vi "Update_Current_Value_client.vi"(0 "Don't Bother with check?":bool, 1 "Update array in":T1[](array[typedef]) {"New Value" format="%.2f"}) -> ()   [LabVIEW 2017]
doc: "This is an example of using features of the VI Server as a client. It shows how you might browse from one or more applications that may be exporting data from one or more data stations. \n\nThe example shows how to query a server for its list of exported VIs, how to get references to the VIs, and how call them with the Call By Reference function."
uses:
  Sub VIs/ADAM Controls/Update_scan_value.ctl
  Anemometry/Anemometry Sub Vis/Controls/Global_mode.ctl
  Anemometry/Anemometry Sub Vis/Globals/Preference_global.vi
panel:
  in  "Server type":refnum<vi>
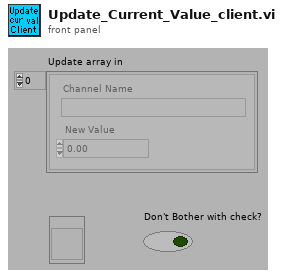
[diagram p1: front panel]
types:
  T1 = typedef "Update_scan_value.ctl" = cluster{"Channel Name":string, "New Value":dbl}
  T2 = typedef "Server_Comms.ctl" = enum16{"Server Link Healthy", "Do Not Link To Server"}
  T3 = typedef "Global_mode.ctl" = enum16{"Read Global", "Load Global From File", "Write Global to File"}
  T4 = enum16{"Append to Global", "Read Global then Clear"}
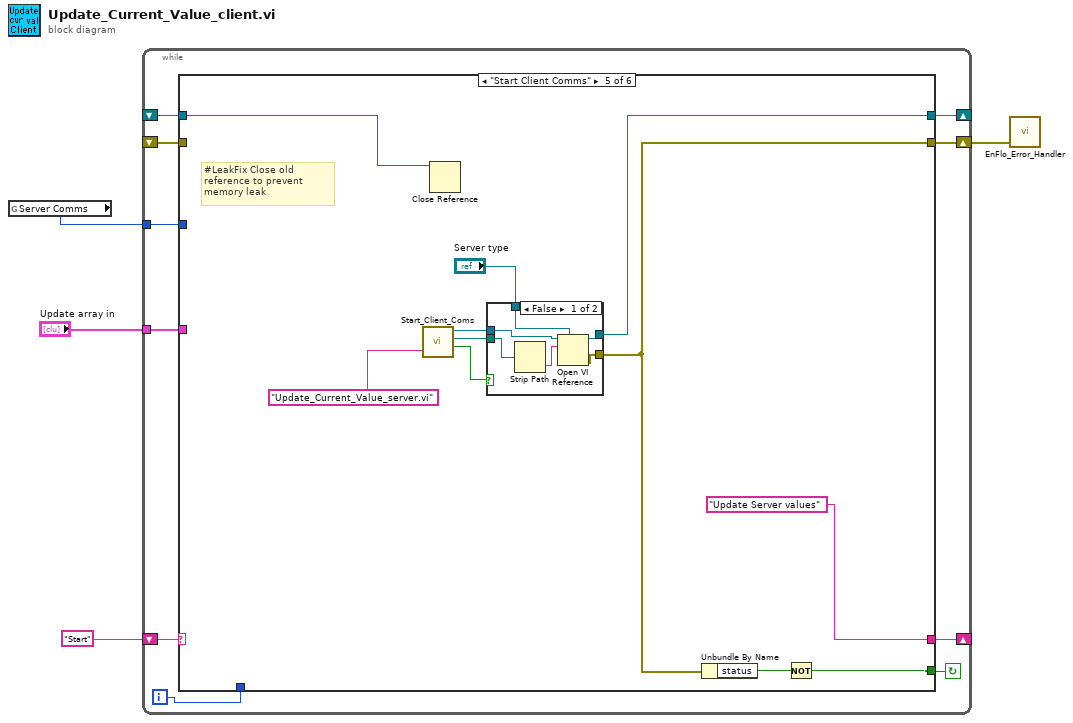
[diagram p0: block diagram]
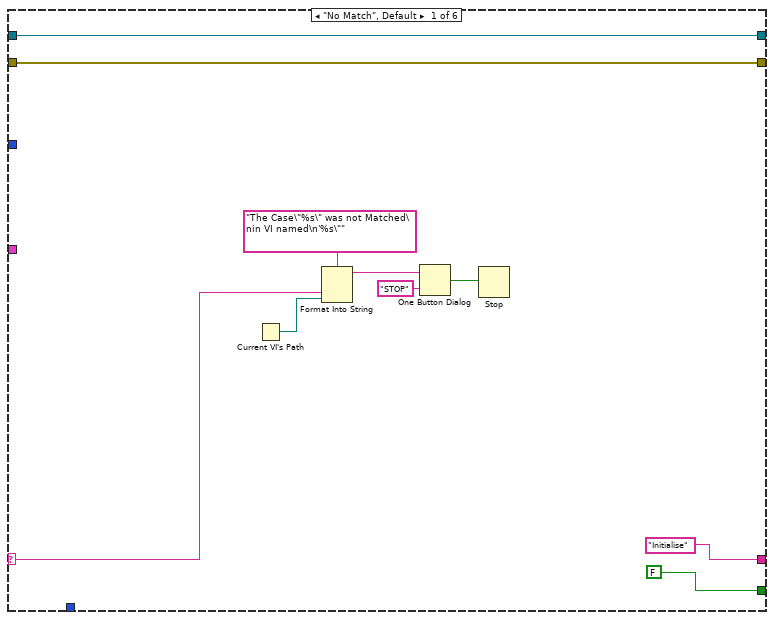
[diagram p2: hidden frame]
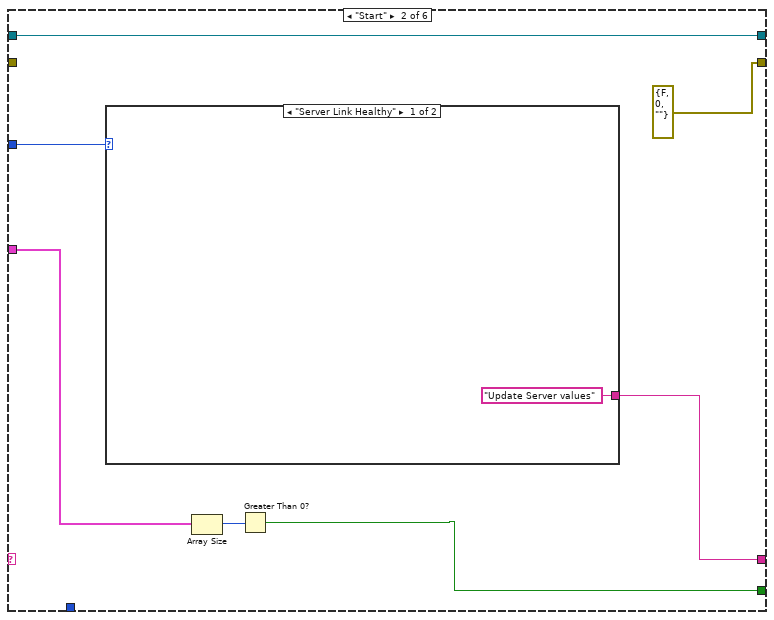
[diagram p3: hidden frame]
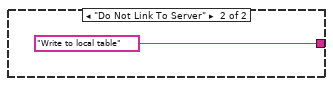
[diagram p4: hidden frame]
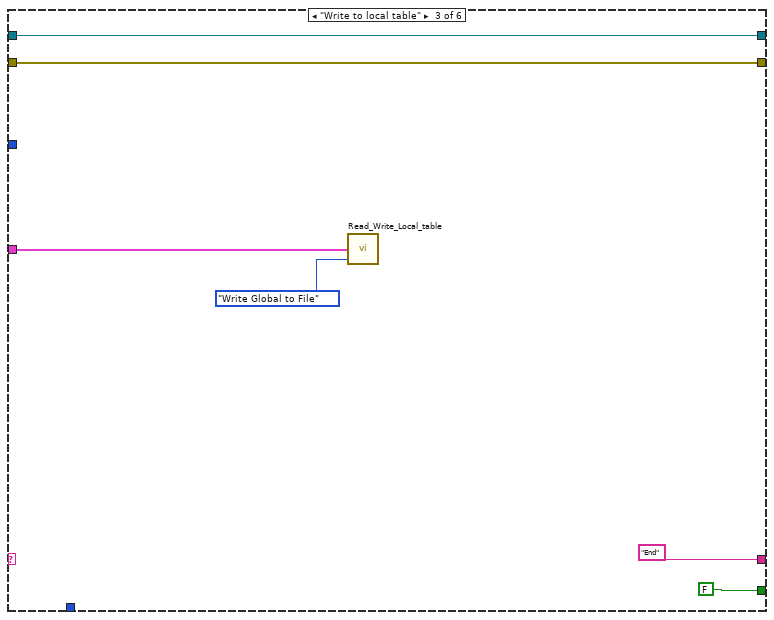
[diagram p5: hidden frame]
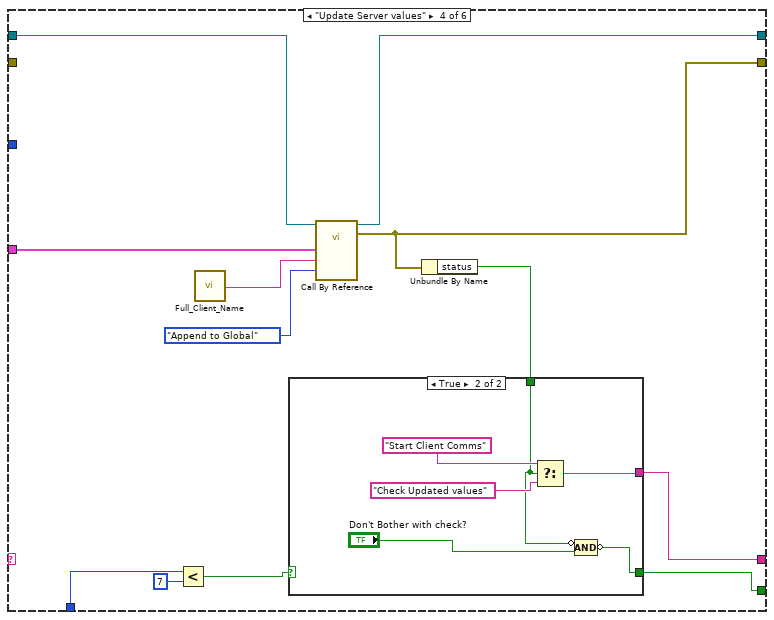
[diagram p6: hidden frame]
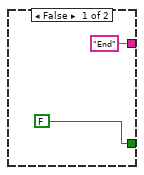
[diagram p7: hidden frame]
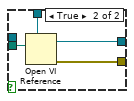
[diagram p8: hidden frame]
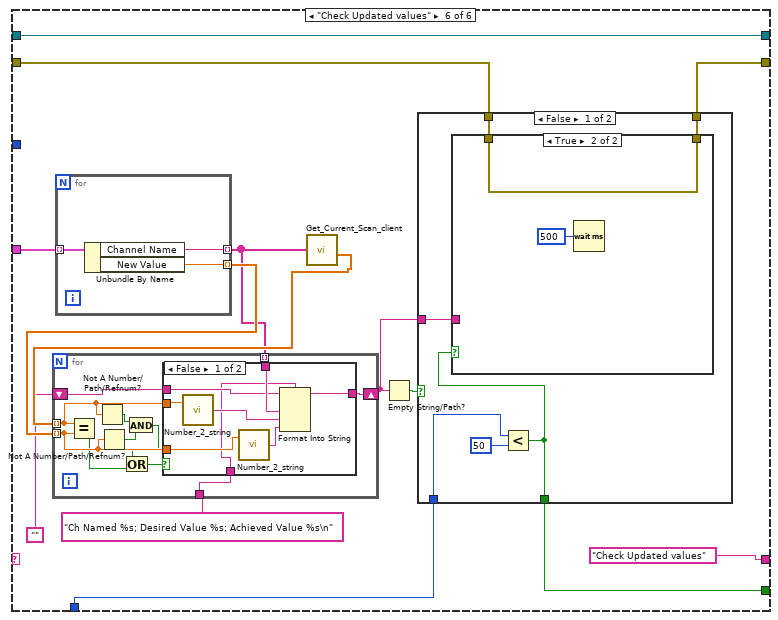
[diagram p9: hidden frame]
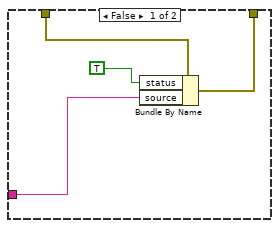
[diagram p11: hidden frame]
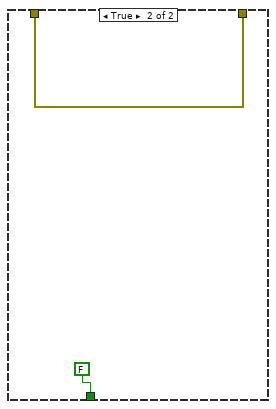
[diagram p12: hidden frame]
diagram:
  n1 = global read "Preference_global.vi" "Server Comms"() -> (w3:T2)
  n2 = while {
    shift-left: "Start" -> [w12]
    shift-right: [w13] -> _
    tunnel: w3 -> [w11]
    tunnel: "Update array in" -> [w10]
    shift-right: [w8] -> _
    shift-left: _ -> [w9]
    shift-right: [w7] -> w1
    shift-left: _ -> [w5]
    i -> [w6]
    stop <- w14 continue-if-true
    n3 = case shown="\"Start Client Comms\"" w12 {
      selector: w12 -> [w15 _ _ _ _ _]
      tunnel: [FALSE w27 FALSE w40 w62 w92] -> w14
      tunnel: ["Initialise" w26 "End" w45 "Update Server values" "Check Updated values"] -> w13
      tunnel: w11 -> [_ w31 _ _ _ _]
      tunnel: w10 -> [_ w29 w36 w49 _ w94]
      tunnel: w9 -> [w17 w30 w35 w47 w60 w93]
      tunnel: [w17 w30 w35 w48 w65 w93] -> w8
      tunnel: [w16 errorcluster {"status"=FALSE, "code"=0, "source"=""} ("Error IO") w34 w44 w64 w82] -> w7
      tunnel: w6 -> [_ _ _ w43 _ w81]
      tunnel: w5 -> [w16 _ w34 _ _ w90]
      frame "No Match", Default {
        n4 = Current VI's Path() -> (path=w19:path)
        n5 = Format Into String(format string="The Case\"%s\" was not Matched\nin VI named\n'%s\"" ("Format String"), w15, w19) -> (resulting string=w22:string)  [unwired: 2 in, 1 out]
        n6 = One Button Dialog(message=w22, button name ("OK")="STOP") -> (true=w20:bool)
        n7 = Stop(stop? (T)=w20) -> ()
      }
      frame "Start" {
        n8 = case shown="\"Server Link Healthy\"" w31 {
          tunnel: ["Update Server values" "Write to local table"] -> w26
          frame "Server Link Healthy" {
          }
          frame "Do Not Link To Server" {
          }
        }
        n9 = Array Size(array=w29) -> (size(s)=w28:i32)
        n10 = Greater Than 0?(x=w28) -> (x > 0?=w27:bool)
      }
      frame "Write to local table" {
        n11 = call "Read_Write_Local_table.vi"("Mode"=Global_mode."Write Global to File", "Ch Values in"=w36) -> ()  [unwired: 1 in, 3 out]
      }
      frame "Update Server values" {
        n12 = Less?(x=w43, y=7) -> (x < y?=w41:bool)
        n13 = call "Full_Client_Name.vi"() -> ("Client Name"=w51:string)
        n14 = call-by-ref "?"(reference=w47, "Mode"=T4."Append to Global", "Client HD name"=w51, "Update array in"=w49) -> (reference out=w48:refnum<vi>, error out=w44:errorcluster)  [unwired: 1 in, 1 out]
        n15 = Unbundle By Name(w44) -> ("status"=w46:bool)
        n16 = case shown="True" w41 {
          tunnel: w46 -> [_ w56]
          tunnel: ["End" w57] -> w45
          tunnel: [FALSE w54] -> w40
          frame False {
          }
          frame True {
            n17 = Select(t="Start Client Comms", s=w56, f="Check Updated values") -> (s? t:f=w57:string)
            n18 = Compound Arithmetic op=AND(invert w56, "Don't Bother with check?") -> (invert w54:bool)
          }
        }
      }
      frame "Start Client Comms" {
        # "#LeakFix Close old reference to prevent memory leak"
        n19 = call "Start_Client_Coms.vi"("VI name to run on server"="Update_Current_Value_server.vi") -> ("LabVIEW application reference"=w68:refnum<vi>, "Checked VI name"=w67:path, "Local Call"=w69:bool)  [unwired: 1 in, 1 out]
        n20 = Close Reference(reference=w60) -> ()  [unwired: 1 in, 1 out]
        n21 = case shown="False" w69 {
          tunnel: [w75 w80] -> w65
          tunnel: "Server type" -> [w73 w79]
          tunnel: w67 -> [w72 w78]
          tunnel: w68 -> [w71 _]
          tunnel: [w74 w77] -> w64
          frame False {
            n22 = Strip Path(path=w72) -> (name=w76:string)  [unwired: 1 out]
            n23 = Open VI Reference(type specifier VI Refnum (for type only)=w73, application reference (local)=w71, vi path=w76) -> (vi reference=w75:refnum<vi>, error out=w74:errorcluster)  [unwired: 1 in, 2 out]
          }
          frame True {
            n24 = Open VI Reference(type specifier VI Refnum (for type only)=w79, vi path=w78) -> (vi reference=w80:refnum<vi>, error out=w77:errorcluster)  [unwired: 1 in, 3 out]
          }
        }
        n25 = Unbundle By Name(w64) -> ("status"=w63:bool)
        n26 = Not(x=w63) -> (.not. x?=w62:bool)
      }
      frame "Check Updated values" {
        n27 = for {
          tunnel: w94 -> [w131] mode=indexing
          tunnel: [w130] -> w87 mode=indexing
          tunnel: [w129] -> w89 mode=indexing
          n28 = Unbundle By Name(w131) -> ("Channel Name"=w130:string, "New Value"=w129:dbl)
        }
        n29 = call "Get_Current_Scan_client.vi"("ADAM Ch Names"=w87) -> ("Numerical Values"=w88:dbl[])  [unwired: 3 out]
        n30 = for {
          shift-right: [w103] -> w83
          shift-left: "" -> [w102]
          tunnel: w89 -> [w99] mode=indexing
          tunnel: w88 -> [w100] mode=indexing
          tunnel: w87 -> [w105] mode=indexing
          tunnel: "Ch Named %s; Desired Value %s; Achieved Value %s\n" ("format string") -> [w104]
          n31 = Equal?(x=w100, y=w99) -> (x = y?=w95:bool)
          n32 = Not A Number/Path/Refnum?(number/path/refnum=w100) -> (NaN/Path/Refnum?=w97:bool)
          n33 = Not A Number/Path/Refnum?(number/path/refnum=w99) -> (NaN/Path/Refnum?=w98:bool)
          n34 = And(x=w97, y=w98) -> (x .and. y?=w96:bool)
          n35 = Or(x=w96, y=w95) -> (x .or. y?=w101:bool)
          n36 = case shown="False" w101 {
            tunnel: w105 -> [w113 _]
            tunnel: w100 -> [w107 _]
            tunnel: w99 -> [w108 _]
            tunnel: w104 -> [w106 _]
            tunnel: [w112 w114] -> w103
            tunnel: w102 -> [w111 w114]
            frame False {
              n37 = call "Number_2_string.vi"("number"=w107) -> ("String"=w109:string)  [unwired: 1 in]
              n38 = call "Number_2_string.vi"("number"=w108) -> ("String"=w110:string)  [unwired: 1 in]
              n39 = Format Into String(format string=w106, initial string=w111, w113, w109, w110) -> (resulting string=w112:string)  [unwired: 1 in, 1 out]
            }
            frame True {
            }
          }
        }
        n40 = Empty String/Path?(string/path=w83) -> (empty?=w84:bool)
        n41 = case shown="False" w84 {
          tunnel: [w115 FALSE] -> w92
          tunnel: w90 -> [w120 w127]
          tunnel: w83 -> [w119 _]
          tunnel: [w118 w127] -> w82
          tunnel: w81 -> [w116 _]
          frame False {
            n42 = Less?(x=w116, y=50) -> (x < y?=w115:bool)
            n43 = case shown="True" w115 {
              tunnel: w120 -> [w124 w125]
              tunnel: w119 -> [w122 _]
              tunnel: [w121 w125] -> w118
              frame False {
                n44 = Bundle By Name(cluster=w124, "status"=TRUE, "source"=w122) -> (w121:errorcluster)
              }
              frame True {
                n45 = Wait (ms)(milliseconds to wait=u32 500) -> ()  [unwired: 1 out]
              }
            }
          }
          frame True {
          }
        }
      }
    }
  }
  n46 = call "EnFlo_Error_Handler.vi"("error in (no error)"=w1) -> ()  [unwired: 2 in, 3 out]
